vi "Load Config File (SubVI).vi"() -> (0 "sortie d'erreur":errorcluster, 2 "Type .EXE":bool, 3 "Refnum VISA en sortie":refnum<visa-resource-name>)   [LabVIEW 2017]
doc: "by Tanguy BOULARD"
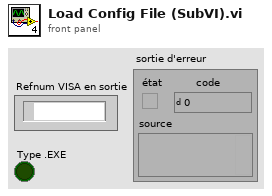
[diagram p1: front panel]
types:
  T1 = enum32{"invalid app kind", "Development System", "Run Time System", "Student Edition", "Embedded LabVIEW", "Evaluation", "Custom"}
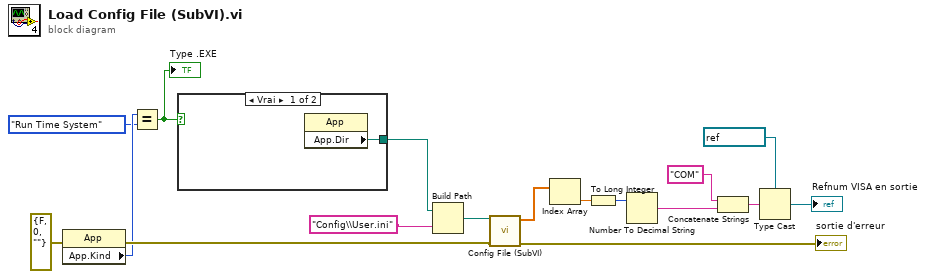
[diagram p0: block diagram]
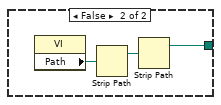
[diagram p2: hidden frame]
diagram:
  n1 = property class="App"(error in=errorcluster {"status"=FALSE, "code"=0, "source"=""} ("error out")) -> (error out=w9:errorcluster, "App.Kind"=w3:T1)  [unwired: 1 in, 1 out]
  n2 = Equal?(x=w3, y=T1."Run Time System" ("Application:Kind")) -> (x = y?=w6:bool)
  "Type .EXE" <- w6
  n3 = case shown="Vrai" w6 {
    tunnel: [w18 w19] -> w7
    frame True {
      n4 = property class="App"() -> ("App.Dir"=w18:path)  [unwired: 2 in, 2 out]
    }
    frame False {
      n5 = property class="VI"() -> ("Path"=w20:path)  [unwired: 2 in, 2 out]
      n6 = Strip Path(path=w20) -> (stripped path=w21:path)  [unwired: 1 out]
      n7 = Strip Path(path=w21) -> (stripped path=w19:path)  [unwired: 1 out]
    }
  }
  n8 = Build Path(base path=w7, name or relative path="Config\\User.ini" ("User_file_name")) -> (appended path=w8:path)
  n9 = call "Config File (SubVI).vi"("entrée d'erreur (pas d'erreur)"=w9, "configuration file path"=w8) -> ("sortie d'erreur"=→"sortie d'erreur":errorcluster, "User file contents"=w15:dbl[])  [unwired: 8 in]
  n10 = Index Array(array=w15) -> (element=w16:dbl)  [unwired: 1 in]
  n11 = To Long Integer(number=w16) -> (32bit integer=w11:i32)
  n12 = Number To Decimal String(number=w11) -> (decimal integer string=w12:string)  [unwired: 1 in]
  n13 = Concatenate Strings("COM" ("string"), w12) -> (w13:string)
  n14 = Type Cast(type=refnum<visa-resource-name> "COM1" ("Com Port"), x=w13) -> (*(type *) &x=→"Refnum VISA en sortie":refnum<visa-resource-name>)
